vi "getAnonymousCredentials.vi"(11 "LocalQueueConnection":refnum<class "LocalQueueConnection.lvclass">) -> (1 "Anonymous password":string, 2 "Anonymous username":string)   [LabVIEW 2013, in "MQTT_Queue.lvlib" / "LocalQueueConnection.lvclass"]
uses:
  LocalQueueConnection.lvclass
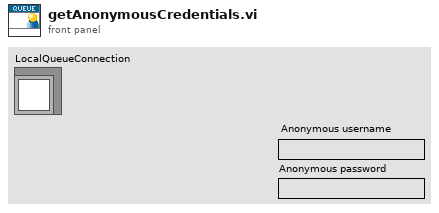
[diagram p1: front panel]
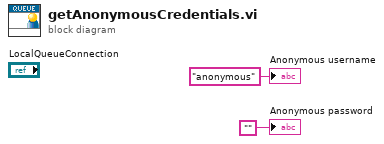
[diagram p0: block diagram]
diagram:
  "Anonymous username" <- "anonymous" ("Anonymous username")
  "Anonymous password" <- ""
